vi "3D-隔行截取法.vi"(11 "原始数据":dbl[][](array[numeric])=array500x800[400000 elements]) -> (3 "隔行截取后的数据":dbl[][](array[numeric]))   [LabVIEW 2011]
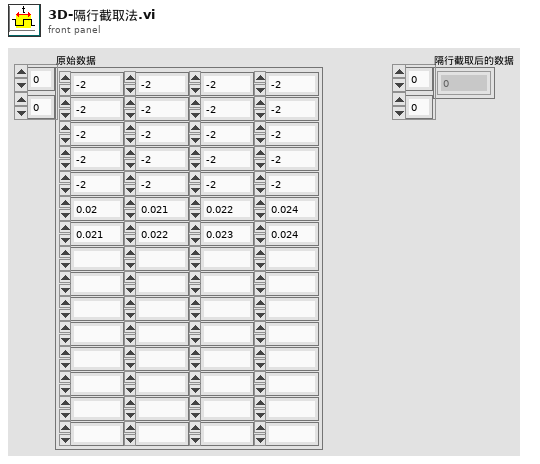
[diagram p1: front panel]
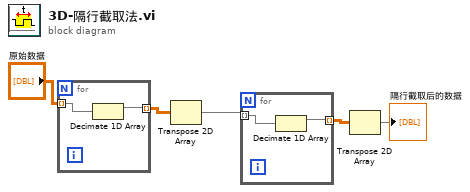
[diagram p0: block diagram]
diagram:
  n1 = for {
    tunnel: "原始数据" -> [w7] mode=indexing
    tunnel: [w6] -> w4 mode=indexing
    n2 = Decimate 1D Array(w7) -> (w6:dbl[])  [unwired: 1 out]
  }
  n3 = Transpose 2D Array(2D array=w4) -> (transposed array=w3:dbl[][])
  n4 = for {
    tunnel: w3 -> [w9] mode=indexing
    tunnel: [w8] -> w2 mode=indexing
    n5 = Decimate 1D Array(w9) -> (w8:dbl[])  [unwired: 1 out]
  }
  n6 = Transpose 2D Array(2D array=w2) -> (transposed array=→"隔行截取后的数据":dbl[][])
